vi "Photon Counting.vi"() -> (13 "Frame acquisition finish?":bool)   [LabVIEW 2015]
uses:
  <vilib>/eio/EIONode/EIONode.xnode
  <vilib>/Platform/TimedLoop/XDataNode/wakeup.ctl
  <vilib>/Platform/TimedLoop/XDataNode/XDNodeRunTimeDep.lvlib
  <vilib>/Platform/TimedLoop/XDataNode/nitl_modes.ctl
  <vilib>/Platform/TimedLoop/XDataNode/timing_clust.ctl
  <vilib>/Platform/TimedLoop/XDataNode/XDataNode.xnode
  <vilib>/rvi/DataTransferAndStorage/Container/XNode/niFpgaContainer.xnode
  Globals/Global Variable_Pixel Clock.vi
  Globals/Global_Sample per Frame.vi
  <vilib>/rvi/Memory/Memory_Emulation/niFpgaMemoryFastEmulationDramWriteAndRequestData.vi
  <vilib>/rvi/Memory/Memory_Emulation/niFpgaMemoryEmulationDramWriteAndRequestData.vi
  <vilib>/rvi/eio/common/nirviEmuTemplateMethod_errors.vi
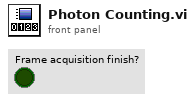
[diagram p1: front panel]
types:
  T1 = typedef "XDNodeRunTimeDep.lvlib/timing_clust.ctl" = cluster{"Expected End [f-1]":u64, "Actual End [f-1]":u64, "Finished Late? [f-1]":bool, "Expected End [i-1]":u64, "Actual End [i-1]":u64, "Finished Late? [i-1]":bool, "Expected Start [i]":u64, "Actual Start [i]":u64, "Expected Start [f]":u64, "Actual Start [f]":u64, "Source Name":string, "Structure Name":string, "Period":i64, "Deadline":i64, "Offset":i64, "Start":i64, "Priority":i32, "Timeout":i32, "Mode":T2, "Wakeup Reason":T3, "Error":errorcluster, "Source Type":string, "Secondary Source Type":string, "Global End Time":u64, "Global Start Time":u64, "Frame Duration":u64, "Iteration Duration":u64, "Assigned CPU":i32, "I/O Scan Engine Mode":u32}
  T2 = typedef "XDNodeRunTimeDep.lvlib/nitl_modes.ctl" = enum32{"No Change", "Process missed periods, maintain original phase", "Discard missed periods, maintain original phase", "Process missed periods, ignore original phase", "Discard missed periods, ignore original phase"}
  T3 = typedef "XDNodeRunTimeDep.lvlib/wakeup.ctl" = enum32{"Normal", "Aborted", "Asynchronous wakeup", "Timing source error", "Timed loop error", "Timeout"}
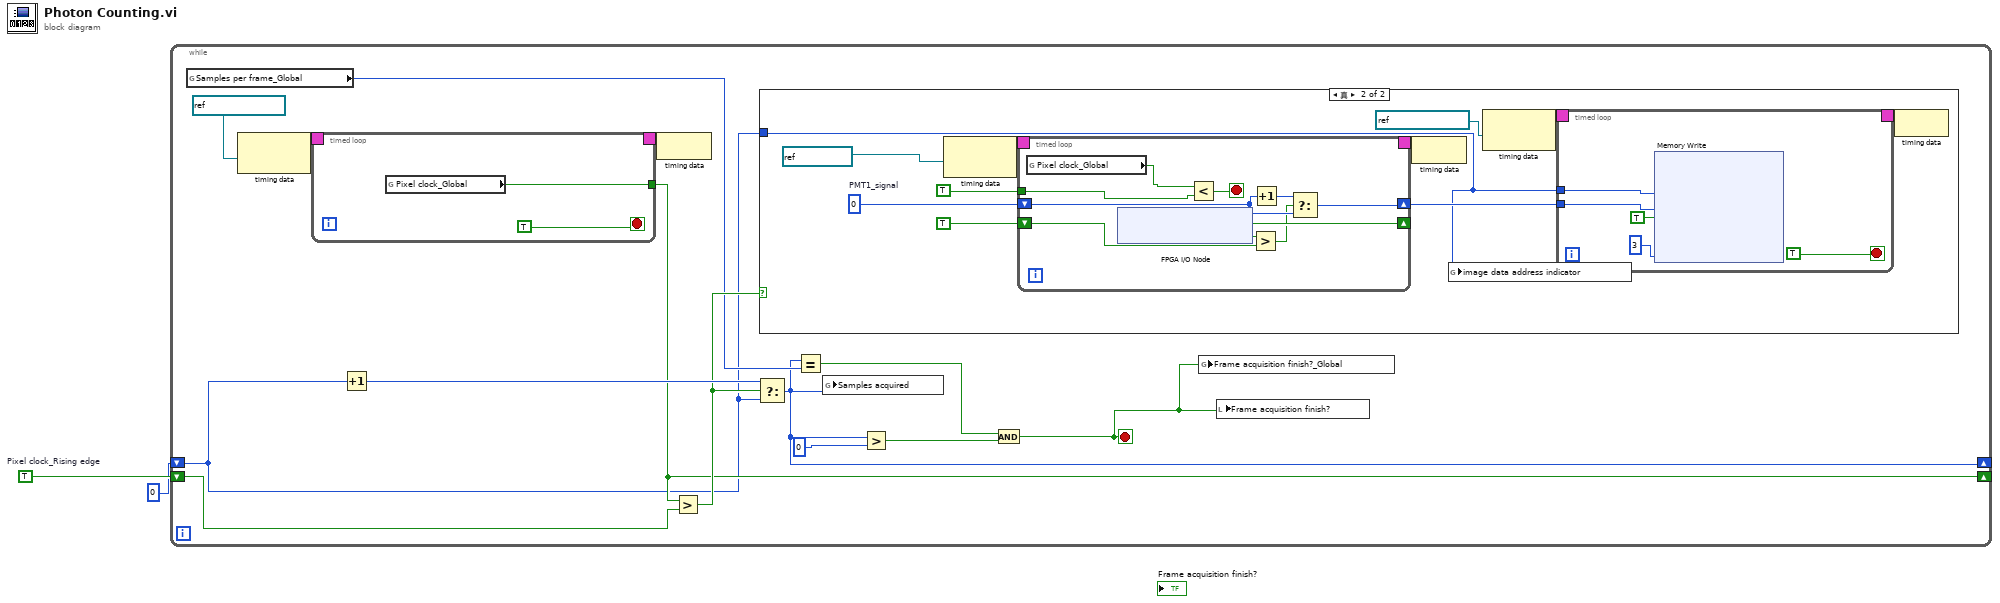
[diagram p0: block diagram]
diagram:
  w2 = TRUE  # Pixel clock_Rising edge
  n1 = while {
    shift-right: [w10] -> _
    shift-left: w2 -> [w12]
    shift-right: [w3] -> _
    shift-left: u32 0 -> [w5]
    stop <- w4 stop-if-true
    n2 = global read "Global_Sample per Frame.vi" "Samples per frame_Global"() -> (w6:u32)
    n3 = node-c288(refnum<k21> "DRAM Clock" ("Source Name")) -> (w9:T1)
    n4 = timed-loop {
      timing: w9 -> [_]
      timing-out: [_] -> w8
      tunnel: [w17] -> w10
      stop <- TRUE stop-if-true
      n5 = global read "Global Variable_Pixel Clock.vi" "Pixel clock_Global"() -> (w17:bool)
    }
    n6 = Increment(x=w5) -> (x+1=w13:u32)
    n7 = node-c288(w8) -> ()
    n8 = Greater?(x=w10, y=w12) -> (0:w11:bool)
    n9 = Select(t=w13, s=w11, f=w5) -> (s? t:f=w3:u32)
    n10 = case shown="真" w11 {
      tunnel: w5 -> [_ w25]
      frame False {
      }
      frame True {
        w33 = u16 0  # PMT1_signal
        n11 = node-c288(refnum<k21> "280MHz" ("Photon counting rate")) -> (w35:T1)
        n12 = timed-loop {
          timing: w35 -> [_]
          timing-out: [_] -> w34
          shift-right: [w53] -> w28
          shift-left: w33 -> [w55]
          shift-right: [w51] -> _
          shift-left: TRUE ("y") -> [w52]
          tunnel: TRUE -> [w49]
          stop <- w48 stop-if-true
          n13 = global read "Global Variable_Pixel Clock.vi" "Pixel clock_Global"() -> (w47:bool)
          n14 = xnode "FPGA I/O Node"() -> ("IO Module\\PMT1"=w51:bool)  [unwired: 1 in, 1 out]
          n15 = Less?(x=w47, y=w49) -> (x < y?=w48:bool)
          n16 = Greater?(x=w51, y=w52) -> (0:w50:bool)
          n17 = Increment(x=w55) -> (x+1=w54:u16)
          n18 = Select(t=w54, s=w50, f=w55) -> (s? t:f=w53:u16)
        }
        n19 = node-c288(w34) -> ()
        n20 = global write "Global_Sample per Frame.vi" "image data address indicator"(w25) -> ()
        n21 = node-c288(refnum<k21> "DRAM Clock" ("Source Name")) -> (w31:T1)
        n22 = timed-loop {
          timing: w31 -> [_]
          timing-out: [_] -> w30
          tunnel: w25 -> [w40]
          tunnel: w28 -> [w39]
          stop <- TRUE stop-if-true
          n23 = xnode ("Memory Write")("地址"=w40, "数据"=w39, "输入有效"=TRUE ("Input Valid"), "字节启用"=i64 3 ("Byte Enables")) -> ()  [unwired: 1 in, 2 out]
        }
        n24 = node-c288(w30) -> ()
      }
    }
    n25 = Equal?(x=w3, y=w6) -> (x = y?=w14:bool)
    n26 = global write "Global_Sample per Frame.vi" "Samples acquired"(w3) -> ()
    n27 = Greater?(x=w3, y=u32 0) -> (0:w15:bool)
    n28 = And(x=w14, y=w15) -> (x .and. y?=w4:bool)
    n29 = global write "Global_Sample per Frame.vi" "Frame acquisition finish?_Global"(w4) -> ()
    n30 = local write "Frame acquisition finish?"(w4) -> ()
  }
